vi "Stop Core.vi"(10 "final error code":i32, 11 "Controller in":refnum<class "Controller.lvclass">) -> (3 "Controller out":refnum<class "Controller.lvclass">)   [LabVIEW 2014, in "Controller.lvlib" / "Controller.lvclass"]
doc: "(<B>Filename</B>: Actor Framework.lvlib:Actor.lvclass:Stop Core.vi)\n\nDefines what the actor does before it stops. Use the <B>final error code</B> input to determine whether the actor shut down in response to an error.\n\nBy default, this method does nothing. A descendant class may override it to define behavior, such as shutting down any processes the actor initiated in its override of the Actor Core method."
uses:
  Controller.lvclass
  reusable/Session APIs/Session Log/System Log.lvclass
  Controls/Notifier Enum.ctl
  reusable/Session APIs/File Access/Config Data/Config Data.lvclass
  Controller.lvclass/Controller.ctl
  reusable/Switch/Switch.lvclass
  <vilib>/ActorFramework/Actor/Actor.lvclass
  <vilib>/NI_Real-Time Target Support.lvlib
  <userlib>/_Session Fwk/Session - Root.lvclass
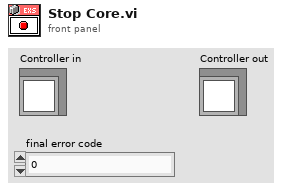
[diagram p1: front panel]
types:
  T1 = typedef "Notifier Enum.ctl" = enum16{"Initialize", "Get", "Set", "Close"}
  T2 = typedef "Session - Root.lvclass/Session Handle.ctl" = refnum<data-value>
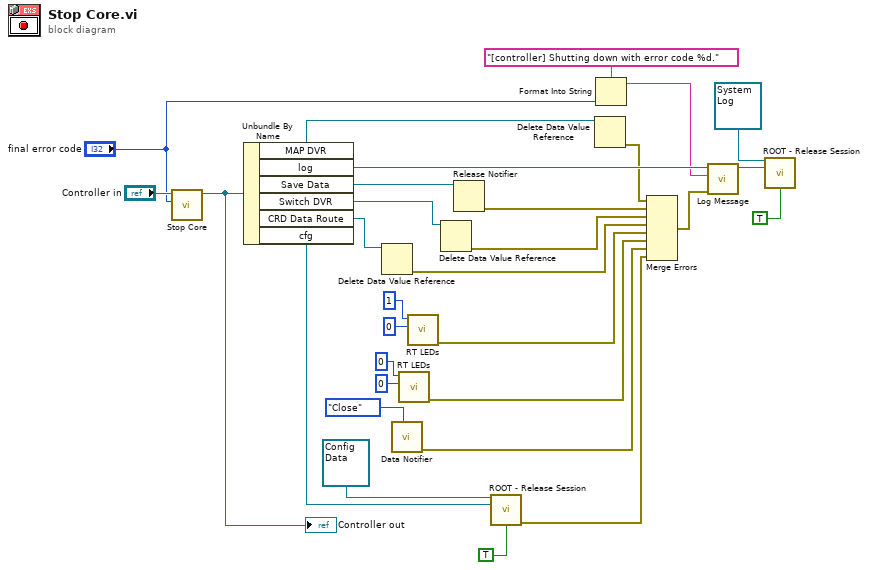
[diagram p0: block diagram]
diagram:
  n1 = call-parent "Stop Core.vi"("final error code"="final error code", "Actor in"="Controller in") -> ("Actor out"=w29:refnum<class "Controller.lvclass">)  [unwired: 9 in]
  "Controller out" <- w29
  n2 = Unbundle By Name(w29) -> ("MAP DVR"=w14:refnum<data-value>, "log"=w27:T2, "Save Data"=w28:refnum<notifier>, "Switch DVR"=w21:refnum<data-value>, "CRD Data Route"=w13:refnum<data-value>, "cfg"=w11:refnum<data-value>)
  n3 = Delete Data Value Reference(data value reference=w13) -> (error out=w1:errorcluster)  [unwired: 1 in, 1 out]
  n4 = call "Data Notifier.vi"("State"=Notifier_Enum."Close") -> ("error out"=w5:errorcluster)  [unwired: 9 in, 1 out]
  n5 = call <vilib>:"RT LEDs.vi"("State"=0, "LED Num"=0) -> ("error out"=w6:errorcluster)  [unwired: 4 in, 1 out]
  n6 = call <vilib>:"RT LEDs.vi"("State"=0 ("LED Num"), "LED Num"=1) -> ("error out"=w2:errorcluster)  [unwired: 4 in, 1 out]
  n7 = Delete Data Value Reference(data value reference=w21) -> (error out=w7:errorcluster)  [unwired: 1 in, 1 out]
  n8 = Release Notifier(notifier=w28) -> (error out=w8:errorcluster)  [unwired: 2 in, 2 out]
  n9 = call <userlib>:"ROOT - Release Session.vi"("OBJ - Session in"=refnum<class "Config Data.lvclass"> refnum ("Config Data"), "Session Handle in"=w11, "force destroy? (F)"=TRUE) -> ("error out"=w4:errorcluster)  [unwired: 11 in, 1 out]
  n10 = Delete Data Value Reference(data value reference=w14) -> (error out=w9:errorcluster)  [unwired: 1 in, 1 out]
  n11 = Format Into String(format string="[controller] Shutting down with error code %d.", "final error code") -> (resulting string=w24:string)  [unwired: 2 in, 1 out]
  n12 = Merge Errors(w9, w8, w7, w1, w2, w6, w5, w4) -> (w3:errorcluster)
  n13 = call "Log Message.vi"("error in"=w3, "MSG In"=w24, "session in"=w27) -> ("session out"=w18:T2)  [unwired: 7 in, 1 out]
  n14 = call <userlib>:"ROOT - Release Session.vi"("OBJ - Session in"=refnum<class "System Log.lvclass"> refnum ("Sys Log"), "Session Handle in"=w18, "force destroy? (F)"=TRUE) -> ()  [unwired: 11 in, 2 out]
